vi "distance2plane.vi"(3 "pt3":dbl[](array[numeric]), 4 "pt2":dbl[](array[numeric]), 5 "pt1":dbl[](array[numeric])) -> (0 "N":dbl[](array[numeric]), 1 "D":dbl, 2 "1/sqrt(A2+B2+C2)":dbl)   [LabVIEW 2021]
uses:
  <vilib>/Analysis/baseanly.llb/Real Dot Product.vi
  <vilib>/Analysis/NI_AALPro.lvlib
  <vilib>/Analysis/NI_AALBase.lvlib
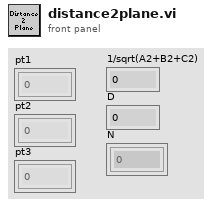
[diagram p1: front panel]
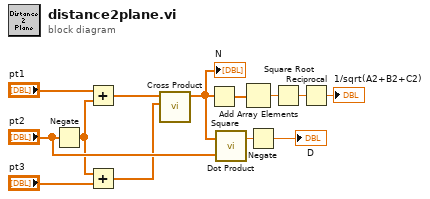
[diagram p0: block diagram]
diagram:
  n1 = Negate(x="pt2") -> (-x=w1:dbl[])
  n2 = Add(x="pt1", y=w1) -> (x+y=w6:dbl[])
  n3 = Add(x=w1, y="pt3") -> (x+y=w7:dbl[])
  n4 = call <vilib>:"Cross Product.vi"("B Vector"=w7, "A Vector"=w6) -> ("Cross Product"=w4:dbl[])  [unwired: 8 in, 1 out]
  "N" <- w4
  n5 = Square(x=w4) -> (x^2=w2:dbl[])
  n6 = call-poly <vilib>:"Dot Product.vi"("Y Vector"="pt2", "X Vector"=w4) -> ("X * Y"=w11:dbl)  [unwired: 1 out]
  n7 = Add Array Elements(numeric array=w2) -> (sum=w3:dbl)
  n8 = Negate(x=w11) -> (-x=→"D":dbl)
  n9 = Square Root(x=w3) -> (sqrt(x)=w10:dbl)
  n10 = Reciprocal(x=w10) -> (1/x=→"1/sqrt(A2+B2+C2)":dbl)
